vi "TcA03-002_ReadingLockingAndSettingClassAttributes.vi"(1 "Input buffer":T3="1", 3 "Invocation info":T2, 5 "error in (no error)":errorcluster, 6 "Add log to result?":bool) -> (16 "Test Data":T1 {"Numeric Measurement" format="%.2f"}, 19 "error out":errorcluster)   [LabVIEW 2009]
doc: "Test case template."
uses:
  Shared/Support_InputBuffer.ctl
  Shared/Support_InvocationInfo.ctl
  Shared/Support_TestData.ctl
  TestClasses/G#BaseClass2_class/G#BaseClass2.lvclass
  <vilib>/addons/_AddQ/G#Object/G#Object.lvclass
  TestClasses/G#SubClass2_class/G#SubClass2.lvclass
  TestClasses/G#BaseClass1_class/G#BaseClass1.lvclass
  TestClasses/G#StaticClass_class/G#StaticClass.lvclass
panel:
  in  "Test name":string="TcA03-002 Reading, locking and setting class attributes"
  out "Test result":bool
  out "Result":string
  # "Verify that class attributes can be locked, read and\nset the attributes and thereby unlock them."
  # "Sub test case"
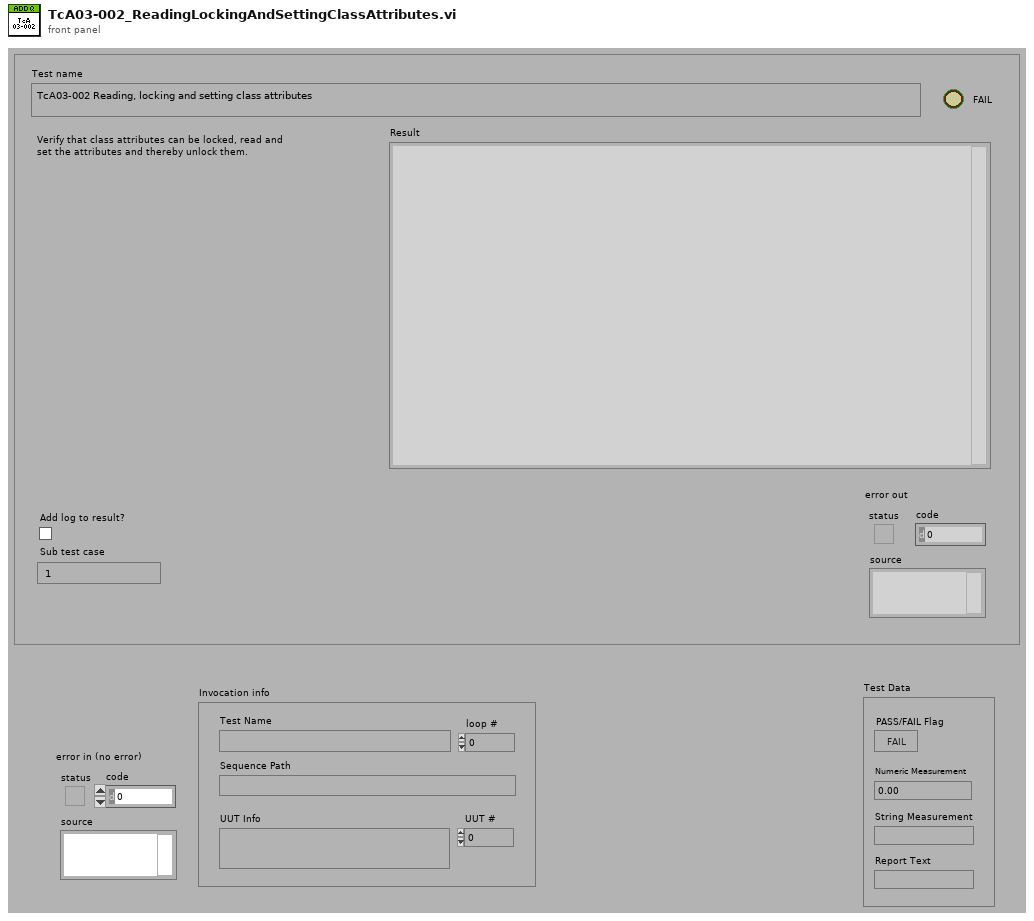
[diagram p1: front panel]
types:
  T1 = typedef "Support_TestData.ctl" = cluster{"PASS/FAIL Flag":bool, "Numeric Measurement":dbl, "String Measurement":string, "Report Text":string}
  T2 = typedef "Support_InvocationInfo.ctl" = cluster{"UUT #":i32, "loop #":i32, "UUT Info":string, "Test Name":string, "Sequence Path":path}
  T3 = typedef "Support_InputBuffer.ctl" = string
  T4 = typedef "Support_ResultType.ctl" = cluster{"Pass":bool, "Comment":string, "MeasurementValue":dbl}
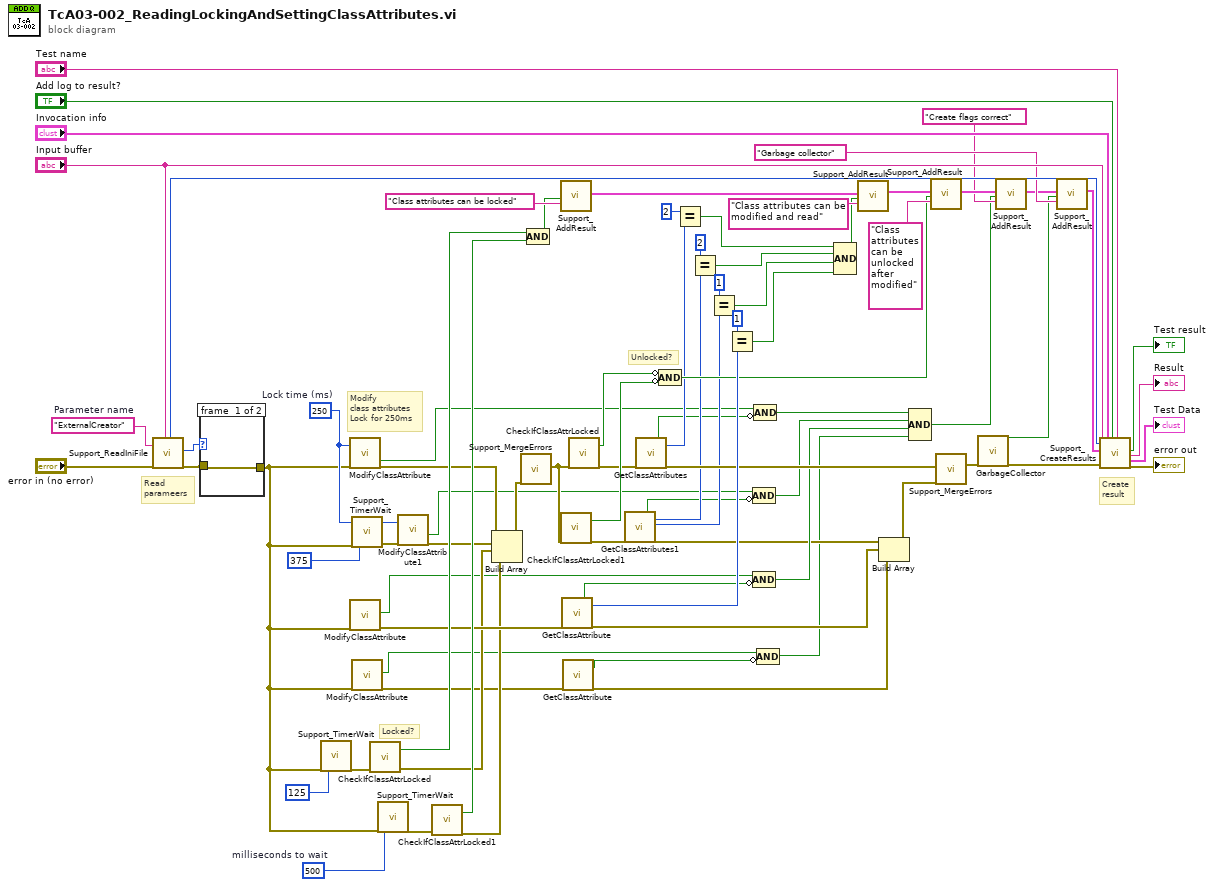
[diagram p0: block diagram]
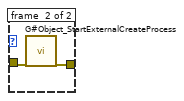
[diagram p2: hidden frame]
diagram:
  w29 = "ExternalCreator"  # Parameter name
  w69 = u32 500  # milliseconds to wait
  w49 = u32 250  # Lock time (ms)
  # "Locked?"
  # "Unlocked?"
  # "Modify\nclass attributes\nLock for 250ms"
  # "Create\nresult"
  # "Read\nparameers"
  n1 = call "Support_ReadIniFile.vi"("Parameter name"=w29, "error in (no error)"="error in (no error)", "Sub test case"="Input buffer") -> ("Timer start"=w72:u32, "Parameter1 as I32"=w27:i32, "error out"=w28:errorcluster)  [unwired: 9 in, 5 out]
  n2 = case shown="1" w27 {
    tunnel: w28 -> [w82 w84]
    tunnel: [w82 w83] -> w9
    frame #0 {
    }
    frame #1 {
      n3 = call <vilib>:"G#Object_StartExternalCreateProcess.vi"("error in (no error)"=w84) -> ("error out"=w83:errorcluster)  [unwired: 18 in]
    }
  }
  n4 = call "Support_TimerWait.vi"("error in (no error)"=w9, "milliseconds to wait"=u32 125) -> ("error out"=w48:errorcluster)  [unwired: 17 in]
  n5 = call "ModifyClassAttribute.vi"("Lock time (ms)"=w49, "error in (no error)"=w9) -> ("created new"=w22:bool, "error out"=w31:errorcluster)  [unwired: 15 in, 1 out]
  n6 = call "ModifyClassAttribute.vi"("error in (no error)"=w9) -> ("created new"=w17:bool, "error out"=w36:errorcluster)  [unwired: 17 in]
  n7 = call "Support_TimerWait.vi"("error in (no error)"=w9, "milliseconds to wait"=u32 375) -> ("error out"=w25:errorcluster)  [unwired: 17 in]
  n8 = call "ModifyClassAttribute.vi"("error in (no error)"=w9) -> ("created new"=w3:bool, "error out"=w8:errorcluster)  [unwired: 17 in]
  n9 = call "CheckIfClassAttrLocked.vi"("error in (no error)"=w48) -> ("locked"=w45:bool, "error out"=w33:errorcluster)  [unwired: 17 in]
  n10 = call "Support_TimerWait.vi"("error in (no error)"=w9, "milliseconds to wait"=w69) -> ("error out"=w47:errorcluster)  [unwired: 17 in]
  n11 = call "ModifyClassAttribute1.vi"("Lock time (ms)"=w49, "error in (no error)"=w25) -> ("created new"=w20:bool, "error out"=w32:errorcluster)  [unwired: 15 in, 1 out]
  n12 = call "CheckIfClassAttrLocked1.vi"("error in (no error)"=w47) -> ("locked"=w46:bool, "error out"=w34:errorcluster)  [unwired: 17 in]
  n13 = Build Array(w31, w32, w33, w34) -> (w30:errorcluster[])
  n14 = call "Support_MergeErrors.vi"("Error array"=w30) -> ("error out"=w35:errorcluster)  [unwired: 17 in, 1 out]
  n15 = Compound Arithmetic op=AND(w45, w46) -> (w66:bool)
  n16 = call "Support_AddResult.vi"("Pass"=w66, "Comment"="Class attributes can be locked") -> ("Results out"=w67:T4[])  [unwired: 17 in]
  n17 = call "CheckIfClassAttrLocked1.vi"("error in (no error)"=w35) -> ("locked"=w42:bool, "error out"=w44:errorcluster)  [unwired: 17 in]
  n18 = call "GetClassAttribute.vi"("error in (no error)"=w36) -> ("created new"=w18:bool, "Int"=w60:i32, "error out"=w6:errorcluster)  [unwired: 15 in, 1 out]
  n19 = call "GetClassAttribute.vi"("error in (no error)"=w8) -> ("created new"=w2:bool, "error out"=w7:errorcluster)  [unwired: 16 in, 1 out]
  n20 = call "CheckIfClassAttrLocked.vi"("error in (no error)"=w35) -> ("locked"=w43:bool, "error out"=w41:errorcluster)  [unwired: 17 in]
  n21 = call "GetClassAttributes1.vi"("error in (no error)"=w44) -> ("created new"=w19:bool, "Base class.ClassAttr"=w38:i32, "SubClassAttr"=w37:i32, "error out"=w5:errorcluster)  [unwired: 15 in]
  n22 = call "GetClassAttributes.vi"("error in (no error)"=w41) -> ("created new"=w21:bool, "ClassAttr"=w39:i32, "error out"=w40:errorcluster)  [unwired: 16 in]
  n23 = Compound Arithmetic op=AND(invert w43, invert w42) -> (w53:bool)
  n24 = Equal?(x=2, y=w39) -> (x = y?=w59:bool)
  n25 = Equal?(x=2, y=w38) -> (x = y?=w58:bool)
  n26 = Equal?(x=1, y=w37) -> (x = y?=w57:bool)
  n27 = Equal?(x=1, y=w60) -> (x = y?=w56:bool)
  n28 = Compound Arithmetic op=AND(w20, invert w19) -> (w11:bool)
  n29 = Compound Arithmetic op=AND(w17, invert w18) -> (w10:bool)
  n30 = Compound Arithmetic op=AND(w22, invert w21) -> (w12:bool)
  n31 = Compound Arithmetic op=AND(w3, invert w2) -> (w1:bool)
  n32 = Compound Arithmetic op=AND(w59, w58, w57, w56) -> (w55:bool)
  n33 = call "Support_AddResult.vi"("Results in"=w67, "Pass"=w55, "Comment"="Class attributes can be modified and read") -> ("Results out"=w23:T4[])  [unwired: 16 in]
  n34 = Build Array(w5, w6, w7) -> (w4:errorcluster[])
  n35 = Compound Arithmetic op=AND(w12, w11, w10, w1) -> (w13:bool)
  n36 = call "Support_AddResult.vi"("Results in"=w23, "Pass"=w53, "Comment"="Class attributes can be unlocked after modified") -> ("Results out"=w16:T4[])  [unwired: 16 in]
  n37 = call "Support_MergeErrors.vi"("error in 1"=w40, "Error array"=w4) -> ("error out"=w71:errorcluster)  [unwired: 16 in, 1 out]
  n38 = call <vilib>:"GarbageCollector.vi"("error in (no error)"=w71) -> ("OK"=w50:bool, "error out"=w70:errorcluster)  [unwired: 16 in, 1 out]
  n39 = call "Support_AddResult.vi"("Results in"=w16, "Pass"=w13, "Comment"="Create flags correct") -> ("Results out"=w15:T4[])  [unwired: 16 in]
  n40 = call "Support_AddResult.vi"("Results in"=w15, "Pass"=w50, "Comment"="Garbage collector") -> ("Results out"=w52:T4[])  [unwired: 16 in]
  n41 = call "Support_CreateResults.vi"("Sub test case"="Input buffer", "Timer start"=w72, "Results"=w52, "error in (no error)"=w70, "Invocation info"="Invocation info", "Add log to result?"="Add log to result?", "Test name"="Test name") -> ("Pass/fail flag"=→"Test result":bool, "Result"=→"Result":string, "Test Data"=→"Test Data":T1, "error out"=→"error out":errorcluster)  [unwired: 9 in]
